vi "Get Message Status.vi"(9 "VI":refnum<vi>, 10 "Actor Class":refnum<vi>, 11 "Message Maker in":refnum<class "Message Maker.lvclass">) -> (1 "Message Type":T1, 3 "Message Status":T2)   [LabVIEW 2023, in "Message Maker.lvclass"]
doc: "Calculates the connector pane, Icon, and description checksum, and compares these to the stored values.\n\nAuthor: Derek Trepanier\nCopyright: MGI 2015"
uses:
  Message Maker.lvclass
  Message Status.ctl
  Message Type.ctl
  Message Maker.lvclass/Message Maker.ctl
  Method Signature.ctl
  <vilib>/LabVIEW Icon API/lv_icon/Classes/Icon/Icon.lvclass
  <vilib>/LabVIEW Icon API/LabVIEW Icon API.lvlib
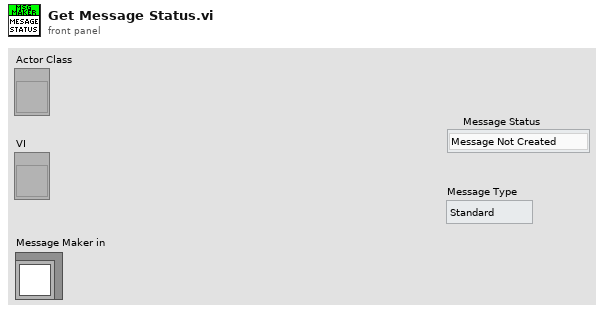
[diagram p1: front panel]
types:
  T1 = typedef "Message Maker.lvclass/Message Type.ctl" = enum16{"Standard", "Async"}
  T2 = typedef "Message Maker.lvclass/Message Status.ctl" = enum16{"Message Not Created", "Message Out of Date", "Message OK", "Never update"}
  T3 = typedef "Message Maker.lvclass/Messages Map.ctl" = map{string, T4}
  T4 = typedef "Message Maker.lvclass/Message Details.ctl" = cluster{"Message Ref":refnum<vi>, "Message Type":T1}
  T5 = typedef "Message Maker.lvclass/Method Signature.ctl" = cluster{"Connector Pane":variant, "Description":string, "Icon":refnum<class "Icon.lvclass">}
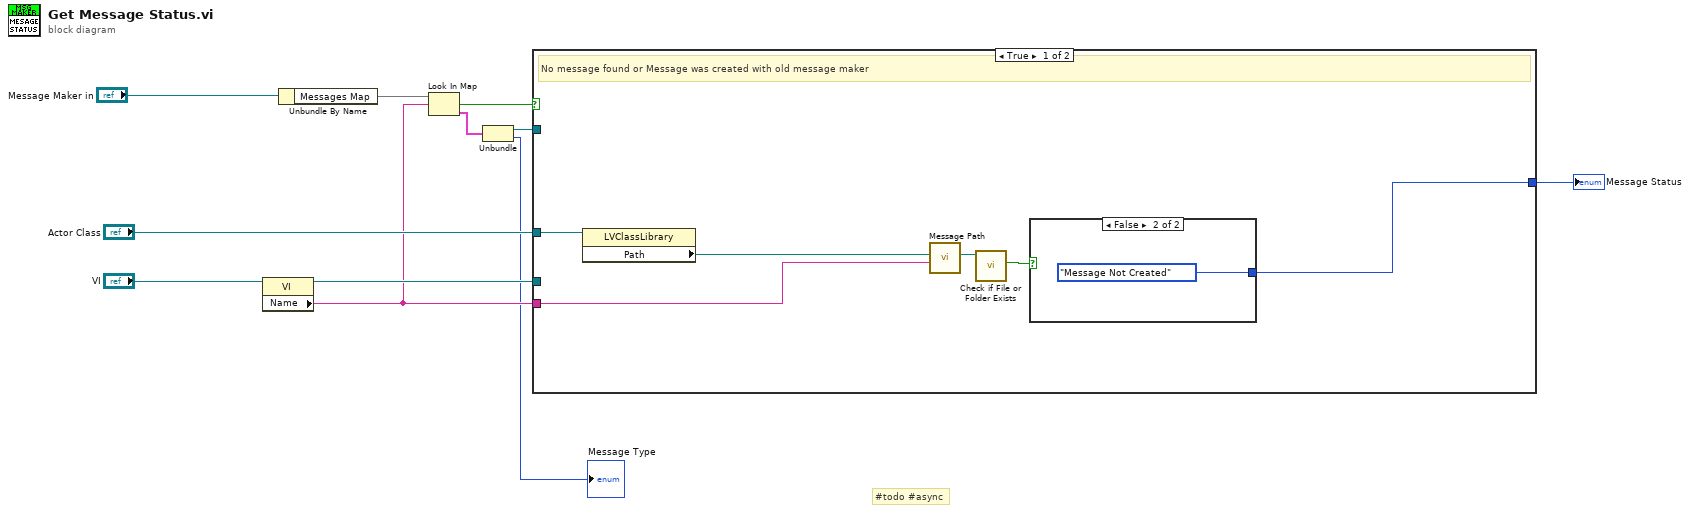
[diagram p0: block diagram]
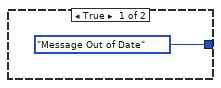
[diagram p2: hidden frame]
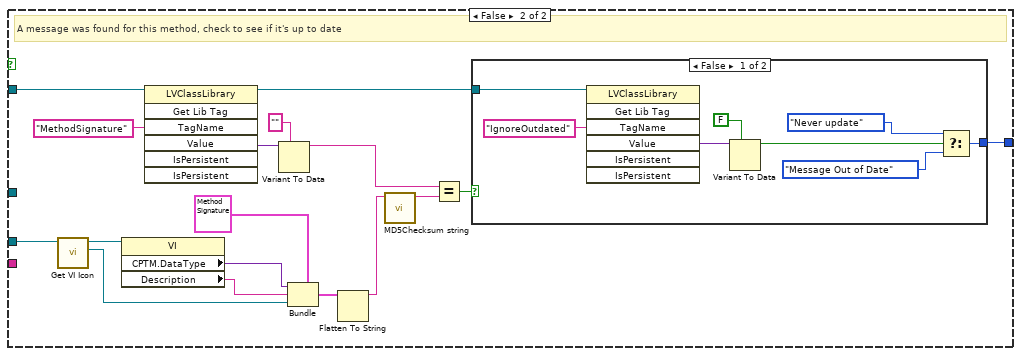
[diagram p3: hidden frame]
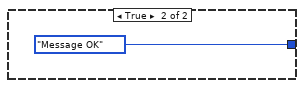
[diagram p4: hidden frame]
diagram:
  # "#todo #async"
  n1 = property class="VI"(reference="VI") -> (reference out=w10:refnum<vi>, "Name"=w5:string)  [unwired: 1 in, 1 out]
  n2 = Unbundle By Name("Message Maker in") -> ("Messages Map"=w6:T3)
  n3 = Look In Map(map=w6, key=w5) -> (key not found?=w4:bool, value=w2:T4)  [unwired: 1 in]
  n4 = Unbundle(w2) -> ("Message Ref"=w3:refnum<vi>, "Message Type"=→"Message Type":T1)
  n5 = case shown="True" w4 {
    tunnel: [w17 w26] -> w11
    tunnel: "Actor Class" -> [w16 _]
    tunnel: w5 -> [w13 _]
    tunnel: w3 -> [_ w36]
    tunnel: w10 -> [_ w34]
    frame True {
      # "No message found or Message was created with old message maker"
      n6 = property class="LVClassLibrary"(reference=w16) -> ("Path"=w15:path)  [unwired: 1 in, 2 out]
      n7 = call "Message Path.vi"("Message Method"=w13, "Class Path"=w15) -> ("Message Class Path"=w14:path)  [unwired: 9 in]
      n8 = call <vilib>:"Check if File or Folder Exists.vi"("path"=w14) -> ("file or folder exists?"=w12:bool)  [unwired: 8 in, 2 out]
      n9 = case shown="False" w12 {
        tunnel: [Message_Status."Message Out of Date" ("Message Status") Message_Status."Message Not Created" ("Message Status")] -> w17
        frame True {
        }
        frame False {
        }
      }
    }
    frame False {
      # "A message was found for this method, check to see if it's up to date"
      n10 = call <vilib>:"Get VI Icon.vi"("VI Refnum in"=w34) -> ("Icon"=w31:refnum<class "Icon.lvclass">, "VI Refnum out"=w33:refnum<vi>)  [unwired: 8 in, 1 out]
      n11 = property class="VI"(reference=w33) -> ("CPTM.DataType"=w32:variant, "Description"=w30:string)  [unwired: 1 in, 2 out]
      n12 = invoke class="LVClassLibrary" method="Get Lib Tag"(reference=w36, "TagName"="MethodSignature" ("Tag Name")) -> (reference out=w20:refnum<vi>, "Value"=w29:variant)  [unwired: 5 in, 5 out]
      n13 = Variant To Data(type="", Variant=w29) -> (data=w28:string)  [unwired: 1 in, 1 out]
      n14 = Bundle(cluster=T5 {"Connector Pane"=variant, "Description"="", "Icon"=refnum} ("output cluster"), "Connector Pane"=w32, "Description"=w30, "Icon"=w31) -> (w24:T5)
      n15 = Flatten To String(anything=w24) -> (data string=w23:string)  [unwired: 3 in, 2 out]
      n16 = call <vilib>:"MD5Checksum string.vi"("Message String"=w23) -> ("MD5 message-digest"=w22:string)  [unwired: 10 in]
      n17 = Equal?(x=w28, y=w22) -> (x = y?=w21:bool)
      n18 = case shown="False" w21 {
        tunnel: [w42 Message_Status."Message OK" ("Message Status")] -> w26
        tunnel: w20 -> [w43 _]
        frame False {
          n19 = invoke class="LVClassLibrary" method="Get Lib Tag"(reference=w43, "TagName"="IgnoreOutdated" ("Tag Name")) -> ("Value"=w39:variant)  [unwired: 5 in, 6 out]
          n20 = Variant To Data(type=FALSE, Variant=w39) -> (data=w38:bool)  [unwired: 1 in, 1 out]
          n21 = Select(t=Message_Status."Never update" ("Message Status"), s=w38, f=Message_Status."Message Out of Date" ("Message Status")) -> (s? t:f=w42:T2)
        }
        frame True {
        }
      }
    }
  }
  "Message Status" <- w11
